vi "savepic.vi"(9 "image data":T1={"image type"=0, "image depth"=8, "image"=array[4584528 elements], "mask"=[], "colors"=[16777215, 16777164, 16777113, 16777062, 16777011, 16776960, 16764159, 16764108, 16764057, 16764006, 16763955, 16763904, 16751103, 16751052, 16751001, 16750950, 16750899, 16750848, 16738047, 16737996, 16737945, 16737894, 16737843, 16737792, 16724991, 16724940, 16724889, 16724838, 16724787, 16724736, 16711935, 16711884, 16711833, 16711782, 16711731, 16711680, 13434879, 13434828, 13434777, 13434726, 13434675, 13434624, 13421823, 13421772, 13421721, 13421670, 13421619, 13421568, 13408767, 13408716, 13408665, 13408614, 13408563, 13408512, 13395711, 13395660, 13395609, 13395558, 13395507, 13395456, 13382655, 13382604, 13382553, 13382502, 13382451, 13382400, 13369599, 13369548, 13369497, 13369446, 13369395, 13369344, 10092543, 10092492, 10092441, 10092390, 10092339, 10092288, 10079487, 10079436, 10079385, 10079334, 10079283, 10079232, 10066431, 10066380, 10066329, 10066278, 10066227, 10066176, 10053375, 10053324, 10053273, 10053222, 10053171, 10053120, 10040319, 10040268, 10040217, 10040166, 10040115, 10040064, 10027263, 10027212, 10027161, 10027110, 10027059, 10027008, 6750207, 6750156, 6750105, 6750054, 6750003, 6749952, 6737151, 6737100, 6737049, 6736998, 6736947, 6736896, 6724095, 6724044, 6723993, 6723942, 6723891, 6723840, 6711039, 6710988, 6710937, 6710886, 6710835, 6710784, 6697983, 6697932, 6697881, 6697830, 6697779, 6697728, 6684927, 6684876, 6684825, 6684774, 6684723, 6684672, 3407871, 3407820, 3407769, 3407718, 3407667, 3407616, 3394815, 3394764, 3394713, 3394662, 3394611, 3394560, 3381759, 3381708, 3381657, 3381606, 3381555, 3381504, 3368703, 3368652, 3368601, 3368550, 3368499, 3368448, 3355647, 3355596, 3355545, 3355494, 3355443, 3355392, 3342591, 3342540, 3342489, 3342438, 3342387, 3342336, 65535, 65484, 65433, 65382, 65331, 65280, 52479, 52428, 52377, 52326, 52275, 52224, 39423, 39372, 39321, 39270, 39219, 39168, 26367, 26316, 26265, 26214, 26163, 26112, 13311, 13260, 13209, 13158, 13107, 13056, 255, 204, 153, 102, 51, 15597568, 14483456, 12255232, 11141120, 8912896, 7798784, 5570560, 4456448, 2228224, 1114112, 60928, 56576, 47872, 43520, 34816, 30464, 21760, 17408, 8704, 4352, 238, 221, 187, 170, 136, 119, 85, 68, 34, 17, 15658734, 14540253, 12303291, 11184810, 8947848, 7829367, 5592405, 4473924, 2236962, 1118481, 0], "Rectangle"={"left"=0, "top"=0, "right"=1488, "bottom"=3081}}, 10 "name":string="NV_switch_dd", 11 "Path":path=path "F:/Tmp" caption="基路径") -> (0 "saved path":path=path "F:/Exp_sum/新建文本文档.txt/NV_switch_dd2018_9_14 13_38_09.jpg", 3 "file name":string="NV_switch_dd2018_9_14 13_38_09")   [LabVIEW 2020]
uses:
  <vilib>/picture/picture.llb/imagedata.ctl
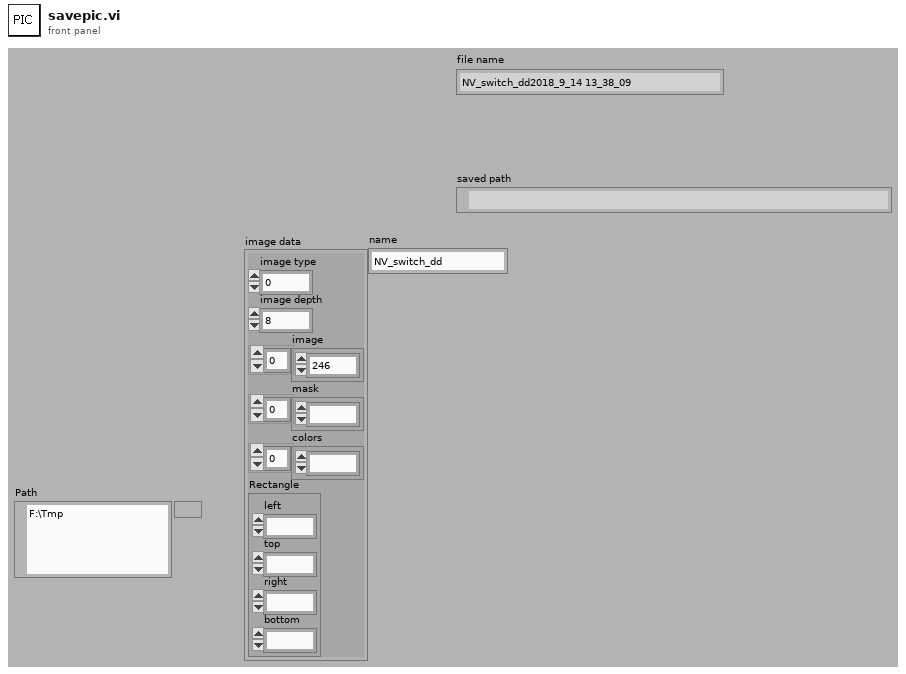
[diagram p1: front panel]
types:
  T1 = typedef "imagedata.ctl" = cluster{"image type":i32, "image depth":i32, "image":u8[], "mask":u8[], "colors":u32[], "Rectangle":cluster{"left":i16, "top":i16, "right":i16, "bottom":i16}}
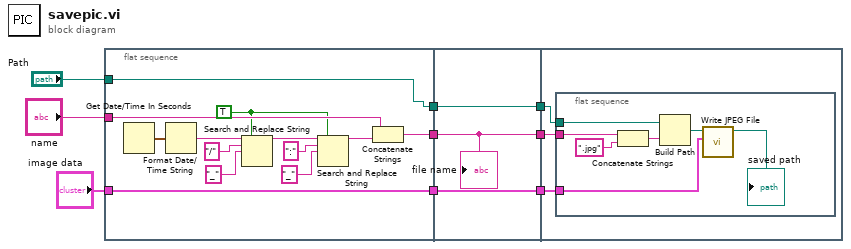
[diagram p0: block diagram]
diagram:
  n1 = flat-sequence {
    tunnel: [w14] -> w9
    tunnel: [w12] -> w8
    tunnel: [w13] -> w4
    tunnel: "image data" -> [w13]
    tunnel: "Path" -> [w12]
    tunnel: "name" -> [w11]
    tunnel: w9 -> [w25]
    tunnel: [w25] -> w7
    tunnel: w8 -> [w24]
    tunnel: [w24] -> w6
    tunnel: [w23] -> w5
    tunnel: w4 -> [w23]
    tunnel: w7 -> [w28]
    tunnel: w6 -> [w27]
    tunnel: w5 -> [w26]
    frame #0 {
      w10 = TRUE ("replace all? (F)")
      n2 = Get Date/Time In Seconds() -> (seconds since 1Jan1904=w16:timestamp)
      n3 = Format Date/Time String(seconds (now)=w16) -> (date/time string=w22:string)  [unwired: 2 in]
      n4 = Search and Replace String(replace all?=w10, input string=w22, search string="/" ("搜索字符串"), replace string="_" ("替换字符串(\"\")")) -> (result string=w19:string)  [unwired: 1 in, 6 out]
      n5 = Search and Replace String(replace all?=w10, input string=w19, search string=":" ("搜索字符串"), replace string="_" ("替换字符串(\"\")")) -> (result string=w15:string)  [unwired: 1 in, 6 out]
      n6 = Concatenate Strings(w11, w15) -> (w14:string)
    }
    frame #1 {
      "file name" <- w25
    }
    frame #2 {
      n7 = flat-sequence {
        tunnel: w28 -> [w34]
        tunnel: w27 -> [w31]
        tunnel: w26 -> [w29]
        frame #0 {
          n8 = Concatenate Strings(w34, ".jpg" ("搜索字符串")) -> (w32:string)
          n9 = Build Path(base path=w31, name or relative path=w32) -> (appended path=w30:path)
          "saved path" <- w30
          n10 = call <vilib>:"Write JPEG File.vi"("image data"=w29, "path to JPEG file"=w30) -> ()  [unwired: 8 in, 2 out]
        }
      }
    }
  }
